vi "Open.vi"(8 "error in (no error)":errorcluster, 10 "Send \"Connect client\"":bool, 11 "RP Communicator in":refnum<class "RP Communicator.lvclass">) -> (0 "error out":errorcluster, 3 "RP Communicator out":refnum<class "RP Communicator.lvclass">)   [LabVIEW 2015, in "RP Communicator.lvclass"]
uses:
  RP Communicator.lvclass
  RP Communicator.lvclass/RP Communicator.ctl
  RP Command.ctl
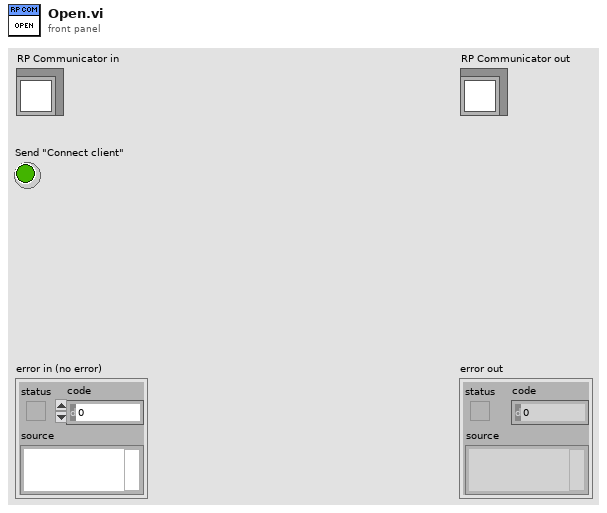
[diagram p1: front panel]
types:
  T1 = typedef "RP Command.ctl" = enum16{"Reset", "Read IDN", "Stop server", "Get status", "Get temperature", "Connect client", "Arm", "Software trigger", "Get whole buffer", "Get chunk", "System call", "Get config", "Set config", "Recieve data", "Play pattern", "Transmit data"}
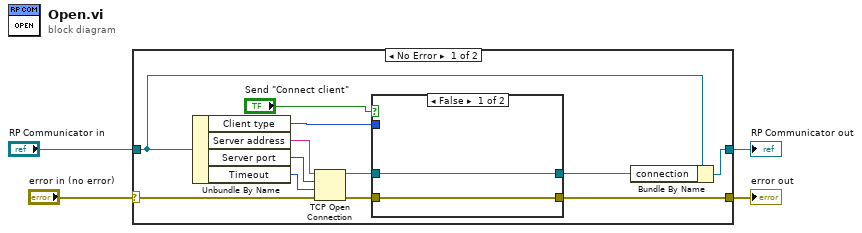
[diagram p0: block diagram]
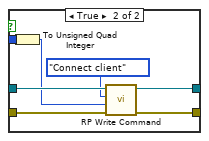
[diagram p2: hidden frame]
diagram:
  n1 = case shown="No Error" "error in (no error)" {
    selector: "error in (no error)" -> [w14 w27]
    tunnel: [w6 w27] -> w3
    tunnel: [w8 w26] -> w1
    tunnel: "RP Communicator in" -> [w9 w26]
    frame No Error {
      n2 = Unbundle By Name(w9) -> ("Client type"=w10:enum16{"Control", "Reciever", "Transmitter"}, "Server address"=w16:string, "Server port"=w15:u16, "Timeout"=w13:i32)
      n3 = TCP Open Connection(address=w16, remote port or service name=w15, timeout ms (60000)=w13, error in (no error)=w14) -> (connection ID=w11:refnum<k5>, error out=w12:errorcluster)  [unwired: 1 in]
      n4 = case shown="False" "Send \"Connect client\"" {
        tunnel: w12 -> [w17 w25]
        tunnel: w11 -> [w18 w24]
        tunnel: w10 -> [_ w22]
        tunnel: [w18 w20] -> w7
        tunnel: [w17 w19] -> w6
        frame False {
        }
        frame True {
          n5 = To Unsigned Quad Integer(1:w22) -> (0:w21:u64)
          n6 = call "RP Write Command.vi"("Error In"=w25, "Command payload"=w21, "Command number"=RP_Command."Connect client", "connection ID"=w24) -> ("Error Out"=w19:errorcluster, "connection ID out"=w20:refnum<k5>)  [unwired: 5 in, 1 out]
        }
      }
      n7 = Bundle By Name(cluster=w9, "connection"=w7) -> (w8:refnum<class "RP Communicator.lvclass">)
    }
    frame Error {
    }
  }
  "error out" <- w3
  "RP Communicator out" <- w1
